vi "CentralStorage.GetReference.vi"(8 "Error in":errorcluster) -> (0 "Error out":errorcluster, 3 "CentralStorage":refnum<data-value>)   [LabVIEW 2016, in "CentralStorage.lvclass"]
uses:
  CentralStorage.lvclass
  ObjectHandler/ObjectHandler.GetObjectWType.ctl
  ObjectHandler/ObjectHandler.ObjectWType.ctl
  ObjectHandler/ObjectHandler.ObjectType.ctl
  ObjectHandler/ObjectHandler.lvclass
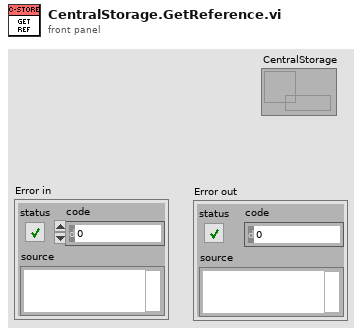
[diagram p1: front panel]
types:
  T1 = typedef "ObjectHandler.lvclass/ObjectHandler.GetObjectWType.ctl" = cluster{"Name":string, "Caller":string}
  T2 = typedef "ObjectHandler.lvclass/ObjectHandler.ObjectWType.ctl" = cluster{"ObjectType":T3, "Object":variant}
  T3 = typedef "ObjectHandler.lvclass/ObjectHandler.ObjectType.ctl" = enum16{"undefined", "ObjectHandler", "ViHandler", "ErrorHandler", "CentralStorage", "Hausmodell", "Sondenmodell", "Wärmepumpe", "Umgebung"}
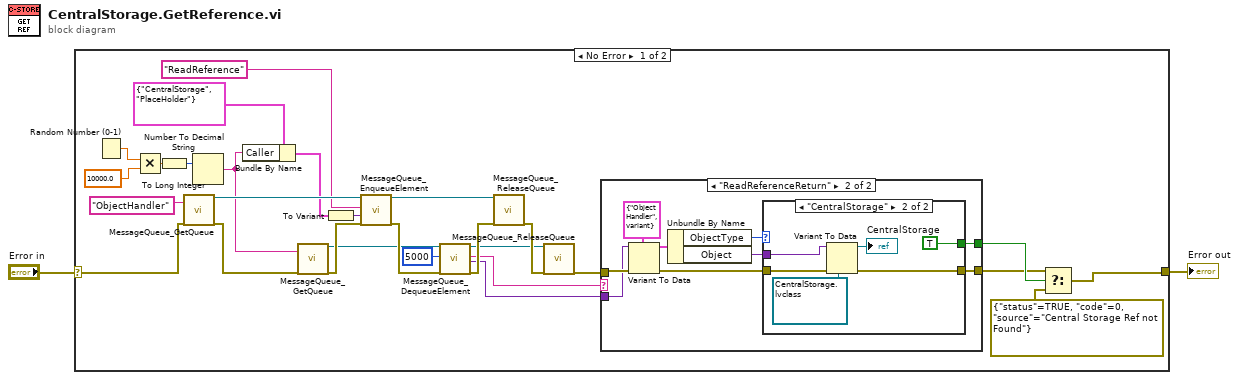
[diagram p0: block diagram]
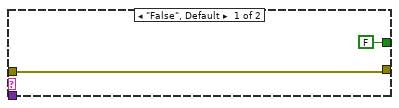
[diagram p2: hidden frame]
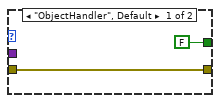
[diagram p3: hidden frame]
diagram:
  n1 = case shown="No Error" "Error in" {
    selector: "Error in" -> [w21 w50]
    tunnel: [w4 w50] -> w2
    frame No Error {
      n2 = Random Number (0-1)() -> (number: 0 to 1=w30:dbl)
      n3 = Multiply(x=w30, y=10000.0) -> (x*y=w28:dbl)
      n4 = To Long Integer(number=w28) -> (32bit integer=w27:i32)
      n5 = call "MessageQueue_GetQueue.vi"("Name"="ObjectHandler", "ErrorIn"=w21) -> ("QueueOut"=w19:refnum<queue>, "ErrorOut"=w22:errorcluster)  [unwired: 15 in, 1 out]
      n6 = Number To Decimal String(number=w27) -> (decimal integer string=w8:string)  [unwired: 1 in]
      n7 = Bundle By Name(cluster=T1 {"Name"="CentralStorage", "Caller"="PlaceHolder"} ("GetRefInput"), "Caller"=w8) -> (w7:T1)
      n8 = call "MessageQueue_GetQueue.vi"("Name"=w8, "ErrorIn"=w22) -> ("QueueOut"=w17:refnum<queue>, "ErrorOut"=w26:errorcluster)  [unwired: 15 in, 1 out]
      n9 = To Variant(anything=w7) -> (Variant=w12:variant)
      n10 = call "MessageQueue_EnqueueElement.vi"("QueueIn"=w19, "Message"="ReadReference", "Data"=w12, "ErrorIn"=w26) -> ("QueueOut"=w18:refnum<queue>, "ErrorOut"=w25:errorcluster)  [unwired: 14 in]
      n11 = call "MessageQueue_DequeueElement.vi"("QueueIn"=w17, "Timeout"=5000, "ErrorIn"=w25) -> ("QueueOut"=w16:refnum<queue>, "Message"=w14:string, "Data"=w10:variant, "ErrorOut"=w24:errorcluster)  [unwired: 12 in, 1 out]
      n12 = call "MessageQueue_ReleaseQueue.vi"("QueueIn"=w18, "ErrorIn"=w24) -> ("ErrorOut"=w23:errorcluster)  [unwired: 15 in, 2 out]
      n13 = call "MessageQueue_ReleaseQueue.vi"("QueueIn"=w16, "ErrorIn"=w23) -> ("ErrorOut"=w11:errorcluster)  [unwired: 15 in, 2 out]
      n14 = case shown="\"ReadReferenceReturn\"" w14 {
        tunnel: w11 -> [w31 w41]
        tunnel: w10 -> [_ w40]
        tunnel: [w31 w34] -> w5
        tunnel: [FALSE w33] -> w6
        frame "False", Default {
        }
        frame "ReadReferenceReturn" {
          n15 = Variant To Data(error in=w41, type=T2 {"ObjectType"=enum."ObjectHandler", "Object"=variant} ("ObjectWType"), Variant=w40) -> (data=w38:T2, error out=w35:errorcluster)
          n16 = Unbundle By Name(w38) -> ("ObjectType"=w37:T3, "Object"=w36:variant)
          n17 = case shown="\"CentralStorage\"" w37 {
            tunnel: w36 -> [_ w49]
            tunnel: w35 -> [w43 w48]
            tunnel: [w43 w47] -> w34
            tunnel: [FALSE TRUE] -> w33
            frame "ObjectHandler", Default {
            }
            frame "CentralStorage" {
              n18 = Variant To Data(error in=w48, type=refnum<data-value> refnum ("data value reference"), Variant=w49) -> (data=→"CentralStorage":refnum<data-value>, error out=w47:errorcluster)
            }
          }
        }
      }
      n19 = Select(t=w5, s=w6, f=errorcluster {"status"=TRUE, "code"=0, "source"="Central Storage Ref not Found"}) -> (s? t:f=w4:errorcluster)
    }
    frame Error {
    }
  }
  "Error out" <- w2
